vi "OE1022D_Reset.vi"(0 "VISA resource name":refnum<visa-resource-name>, 5 "错误输入（无错误）":errorcluster) -> (14 "VISA resource name out":refnum<visa-resource-name>, 19 "错误输出":errorcluster)   [LabVIEW 2014]
doc: "Configures the reference source and the internal oscillator."
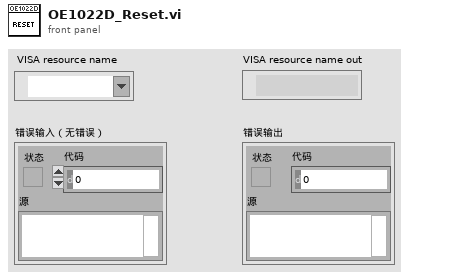
[diagram p1: front panel]
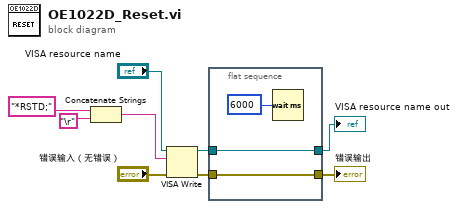
[diagram p0: block diagram]
diagram:
  n1 = Concatenate Strings("*RSTD;" ("string (\"\")"), "\r") -> (w7:string)
  n2 = VISA Write(VISA resource name="VISA resource name", write buffer=w7, error in (no error)="错误输入（无错误）") -> (VISA resource name out=w5:refnum<visa-resource-name>, error out=w3:errorcluster)  [unwired: 1 out]
  n3 = flat-sequence {
    tunnel: [w11] -> w4
    tunnel: w5 -> [w11]
    tunnel: w3 -> [w10]
    tunnel: [w10] -> w2
    frame #0 {
      n4 = Wait (ms)(milliseconds to wait=u32 6000 ("等待时间（毫秒）")) -> ()  [unwired: 1 out]
    }
  }
  "VISA resource name out" <- w4
  "错误输出" <- w2
